vi "Measure.vi"(0 "NI-DMM in":refnum<class "NI-DMM.lvclass">, 11 "error in (no error)":errorcluster) -> (4 "NI-DMM out":refnum<class "NI-DMM.lvclass">, 6 "Measure_Results":variant, 15 "error out":errorcluster)   [LabVIEW 2020, in "AbstractDMM.lvlib" / "NI-DMM.lvclass"]
uses:
  NI-DMM.lvclass
  NI-DMM.lvclass/NI-DMM.ctl
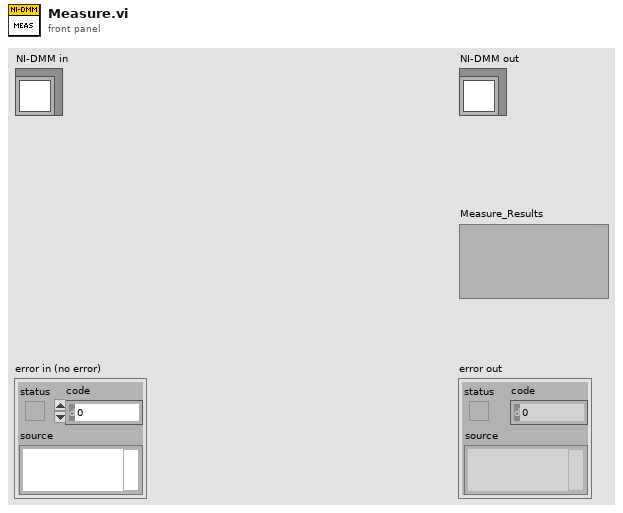
[diagram p1: front panel]
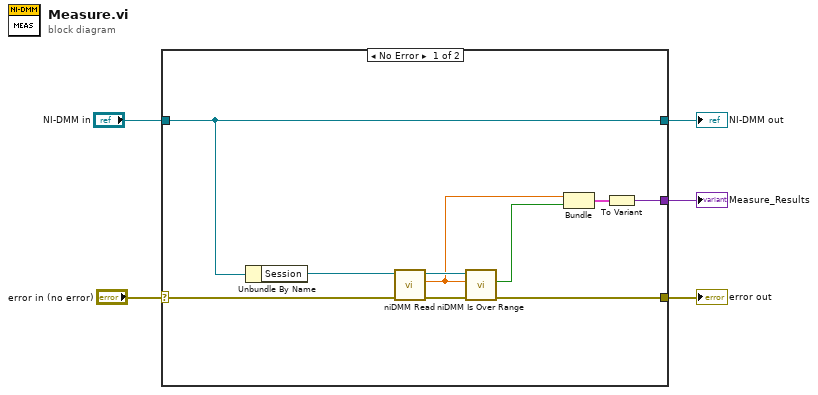
[diagram p0: block diagram]
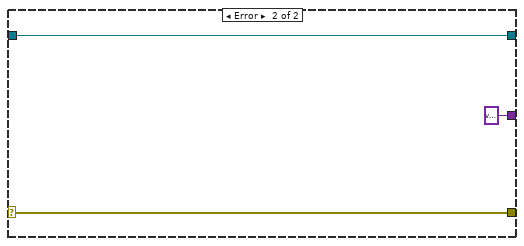
[diagram p2: hidden frame]
diagram:
  n1 = case shown="No Error" "error in (no error)" {
    selector: "error in (no error)" -> [w14 w16]
    tunnel: [w13 w16] -> w4
    tunnel: "NI-DMM in" -> [w6 w18]
    tunnel: [w7 variant ("Variant")] -> w2
    tunnel: [w6 w18] -> w1
    frame No Error {
      n2 = Unbundle By Name(w6) -> ("Session"=w12:refnum<k15>)
      n3 = call <instrlib>:"niDMM Read.vi"("error in (no error)"=w14, "instrument handle"=w12) -> ("error out"=w15:errorcluster, "Measurement"=w10:dbl, "instrument handle out"=w11:refnum<k15>)  [unwired: 7 in]
      n4 = call <instrlib>:"niDMM Is Over Range.vi"("error in (no error)"=w15, "Measurement"=w10, "instrument handle"=w11) -> ("error out"=w13:errorcluster, "Over Range?"=w9:bool)  [unwired: 6 in, 1 out]
      n5 = Bundle("Measurement"=w10, "Over Range?"=w9) -> (w8:cluster{"Measurement":dbl, "Over Range?":bool})  [unwired: 1 in]
      n6 = To Variant(anything=w8) -> (Variant=w7:variant)
    }
    frame Error {
    }
  }
  "error out" <- w4
  "NI-DMM out" <- w1
  "Measure_Results" <- w2
